vi "getCalibrationFromXML.vi"(8 "error in (no error)":errorcluster, 9 "xmlPath":string, 10 "channel_configXML":refnum<class "NativeXML.lvclass">, 11 "RfOutputChannel in":refnum<class "RfOutputChannel.lvclass">) -> (0 "error out":errorcluster, 2 "channel_configXML":refnum<class "NativeXML.lvclass">, 3 "RfOutputChannel out":refnum<class "RfOutputChannel.lvclass">)   [LabVIEW 2011, in "Tools.lvlib" / "DatabaseHelpers.lvlib" / "RfOutputChannel.lvclass"]
uses:
  RfOutputChannel.lvclass
  NativeXML/NativeXML.lvclass
  RfOutputChannel.lvclass/RfOutputChannel.ctl
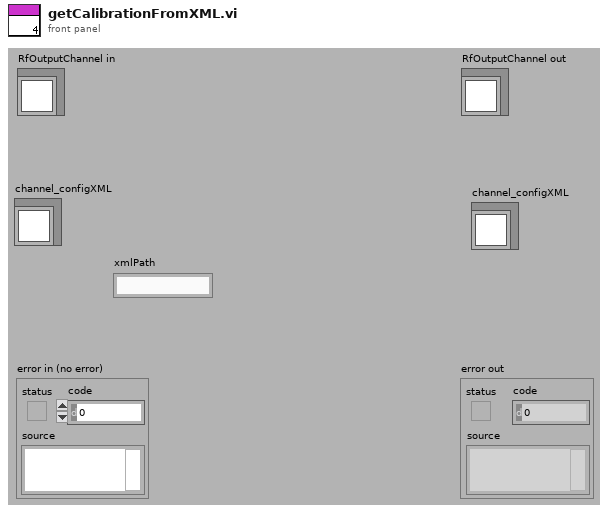
[diagram p1: front panel]
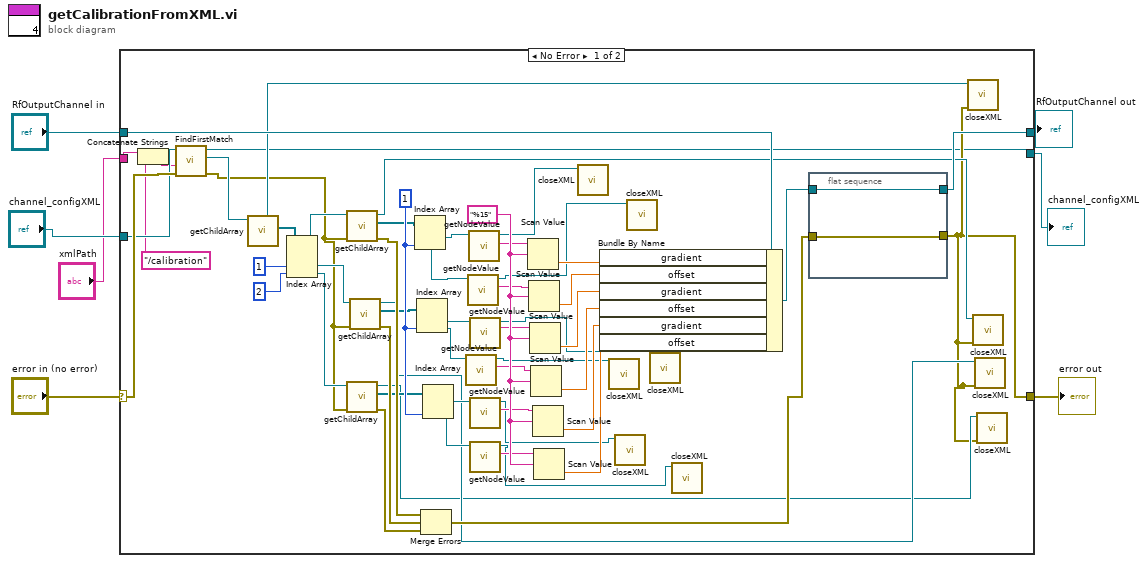
[diagram p0: block diagram]
diagram:
  n1 = case shown="No Error" "error in (no error)" {
    selector: "error in (no error)" -> [w12 w66]
    tunnel: [w18 w66] -> w3
    tunnel: [w23 w65] -> w6
    tunnel: "RfOutputChannel in" -> [w54 w65]
    tunnel: "channel_configXML" -> [w11 _]
    tunnel: [w15 _] -> w2
    tunnel: "xmlPath" -> [w10 _]
    frame No Error {
      w61 = "%15"
      w62 = 1
      n2 = Concatenate Strings(w10, "/calibration") -> (w8:string)
      n3 = call "FindFirstMatch.vi"("error in (no error)"=w12, "xPath"=w8, "NativeXML in"=w11) -> ("error out"=w13:errorcluster, "NativeXML match"=w14:refnum<class "NativeXML.lvclass">, "NativeXML out"=w15:refnum<class "NativeXML.lvclass">)  [unwired: 6 in]
      n4 = call "getChildArray.vi"("NativeXML in"=w14) -> ("childArray"=w51:refnum<class "NativeXML.lvclass">[], "NativeXML out"=w25:refnum<class "NativeXML.lvclass">)  [unwired: 8 in, 1 out]
      n5 = Index Array(array=w51, index #2=1, index #3=2) -> (element #1=w49:refnum<class "NativeXML.lvclass">, element #2=w45:refnum<class "NativeXML.lvclass">, element #3=w44:refnum<class "NativeXML.lvclass">)  [unwired: 1 in]
      n6 = call "getChildArray.vi"("error in (no error)"=w13, "NativeXML in"=w49) -> ("error out"=w48:errorcluster, "childArray"=w50:refnum<class "NativeXML.lvclass">[], "NativeXML out"=w21:refnum<class "NativeXML.lvclass">)  [unwired: 7 in]
      n7 = call "getChildArray.vi"("error in (no error)"=w13, "NativeXML in"=w44) -> ("error out"=w43:errorcluster, "childArray"=w42:refnum<class "NativeXML.lvclass">[], "NativeXML out"=w19:refnum<class "NativeXML.lvclass">)  [unwired: 7 in]
      n8 = call "getChildArray.vi"("error in (no error)"=w13, "NativeXML in"=w45) -> ("error out"=w46:errorcluster, "childArray"=w47:refnum<class "NativeXML.lvclass">[], "NativeXML out"=w20:refnum<class "NativeXML.lvclass">)  [unwired: 7 in]
      n9 = Index Array(array=w50, index #2=w62) -> (element #1=w40:refnum<class "NativeXML.lvclass">, element #2=w38:refnum<class "NativeXML.lvclass">)  [unwired: 1 in]
      n10 = Index Array(array=w47, index #2=w62) -> (element #1=w36:refnum<class "NativeXML.lvclass">, element #2=w34:refnum<class "NativeXML.lvclass">)  [unwired: 1 in]
      n11 = Merge Errors(w48, w46, w43) -> (w22:errorcluster)
      n12 = Index Array(array=w42, index #2=w62) -> (element #1=w32:refnum<class "NativeXML.lvclass">, element #2=w30:refnum<class "NativeXML.lvclass">)  [unwired: 1 in]
      n13 = call "getNodeValue.vi"("NativeXML in"=w34) -> ("Value"=w35:string, "NativeXML out"=w26:refnum<class "NativeXML.lvclass">)  [unwired: 8 in, 1 out]
      n14 = call "getNodeValue.vi"("NativeXML in"=w38) -> ("Value"=w39:string, "NativeXML out"=w28:refnum<class "NativeXML.lvclass">)  [unwired: 8 in, 1 out]
      n15 = call "getNodeValue.vi"("NativeXML in"=w40) -> ("Value"=w41:string, "NativeXML out"=w29:refnum<class "NativeXML.lvclass">)  [unwired: 8 in, 1 out]
      n16 = call "getNodeValue.vi"("NativeXML in"=w36) -> ("Value"=w37:string, "NativeXML out"=w27:refnum<class "NativeXML.lvclass">)  [unwired: 8 in, 1 out]
      n17 = call "getNodeValue.vi"("NativeXML in"=w32) -> ("Value"=w33:string, "NativeXML out"=w17:refnum<class "NativeXML.lvclass">)  [unwired: 8 in, 1 out]
      n18 = call "getNodeValue.vi"("NativeXML in"=w30) -> ("Value"=w31:string, "NativeXML out"=w16:refnum<class "NativeXML.lvclass">)  [unwired: 8 in, 1 out]
      n19 = Scan Value(string=w41, format string=w61) -> (value=w60:dbl)  [unwired: 1 in, 1 out]
      n20 = Scan Value(string=w39, format string=w61) -> (value=w59:dbl)  [unwired: 1 in, 1 out]
      n21 = Scan Value(string=w37, format string=w61) -> (value=w55:dbl)  [unwired: 1 in, 1 out]
      n22 = Scan Value(string=w35, format string=w61) -> (value=w56:dbl)  [unwired: 1 in, 1 out]
      n23 = Scan Value(string=w33, format string=w61) -> (value=w57:dbl)  [unwired: 1 in, 1 out]
      n24 = Scan Value(string=w31, format string=w61) -> (value=w58:dbl)  [unwired: 1 in, 1 out]
      n25 = call "closeXML.vi"("NativeXML in"=w29) -> ()  [unwired: 10 in, 1 out]
      n26 = Bundle By Name(cluster=w54, "gradient"=w60, "offset"=w59, "gradient"=w55, "offset"=w56, "gradient"=w57, "offset"=w58) -> (w24:refnum<class "RfOutputChannel.lvclass">)
      n27 = call "closeXML.vi"("NativeXML in"=w26) -> ()  [unwired: 10 in, 1 out]
      n28 = call "closeXML.vi"("NativeXML in"=w17) -> ()  [unwired: 10 in, 1 out]
      n29 = call "closeXML.vi"("NativeXML in"=w28) -> ()  [unwired: 10 in, 1 out]
      n30 = call "closeXML.vi"("NativeXML in"=w27) -> ()  [unwired: 10 in, 1 out]
      n31 = call "closeXML.vi"("NativeXML in"=w16) -> ()  [unwired: 10 in, 1 out]
      n32 = flat-sequence {
        tunnel: w24 -> [w64]
        tunnel: [w64] -> w23
        tunnel: [w63] -> w18
        tunnel: w22 -> [w63]
        frame #0 {
        }
      }
      n33 = call "closeXML.vi"("error in (no error)"=w18, "NativeXML in"=w25) -> ()  [unwired: 9 in, 1 out]
      n34 = call "closeXML.vi"("error in (no error)"=w18, "NativeXML in"=w21) -> ()  [unwired: 9 in, 1 out]
      n35 = call "closeXML.vi"("error in (no error)"=w18, "NativeXML in"=w20) -> ()  [unwired: 9 in, 1 out]
      n36 = call "closeXML.vi"("error in (no error)"=w18, "NativeXML in"=w19) -> ()  [unwired: 9 in, 1 out]
    }
    frame Error {
    }
  }
  "error out" <- w3
  "RfOutputChannel out" <- w6
  "channel_configXML" <- w2
